vi "WILT Cycle Valve.vi"(7 "Number Of Cycles":i32, 8 "Error In":errorcluster, 10 "Channel":string, 11 "VISA Refnum in":refnum<visa-resource-name>) -> (0 "Error Out":errorcluster)   [LabVIEW 2016]
panel:
  in  "Cycle Time (mS)":u32=1000
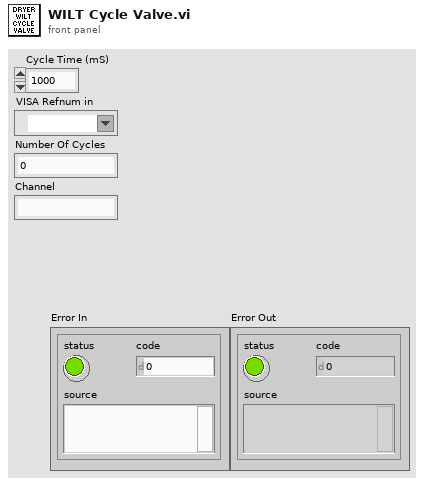
[diagram p1: front panel]
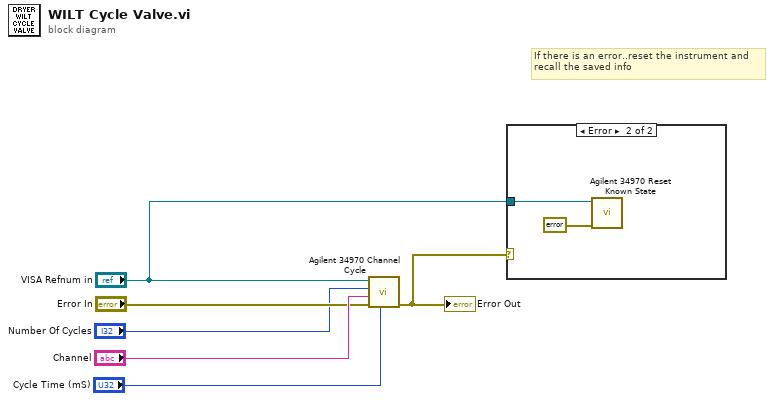
[diagram p0: block diagram]
diagram:
  # "If there is an error..reset the instrument and \nrecall the saved info"
  n1 = call "Agilent 34970 Channel Cycle.vi"("Cycle Time (mS)"="Cycle Time (mS)", "error in (no error)"="Error In", "Channel"="Channel", "Number Of Cycles"="Number Of Cycles", "VISA Refnum in"="VISA Refnum in") -> ("error out"=w3:errorcluster)  [unwired: 5 in, 1 out]
  "Error Out" <- w3
  n2 = case shown="Error" w3 {
    tunnel: "VISA Refnum in" -> [_ w7]
    frame No Error {
    }
    frame Error {
      n3 = call "Agilent 34970 Reset Known State.vi"("Error In"=errorcluster {"status"=TRUE, "code"=0, "source"=""}, "VISA Refnum in"=w7) -> ()  [unwired: 9 in, 1 out]
    }
  }
